vi "Read Events.vi"(8 "error in (no error)":errorcluster, 11 "Engine in":refnum<class "Engine.lvclass">) -> (0 "error out":errorcluster, 2 "Events":T1, 3 "Engine out":refnum<class "Engine.lvclass">)   [LabVIEW 2023, in "Engine.lvlib" / "Engine.lvclass"]
uses:
  Library/Engine.lvclass
  Custom Controls/Events.ctl
  Custom Controls/SystemEvents.ctl
  Custom Controls/Faults.ctl
  Custom Controls/Status.ctl
  Custom Controls/OtherEvents.ctl
  Custom Controls/AbstractMessage.ctl
  Library/Engine.lvclass/Engine.ctl
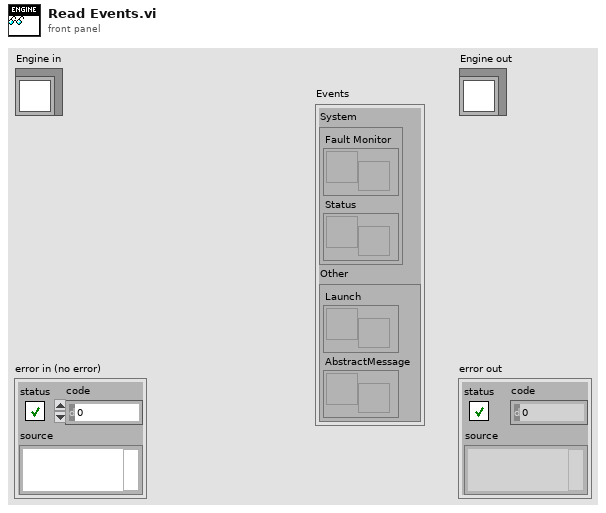
[diagram p1: front panel]
types:
  T1 = typedef "Engine.lvlib/Engine.lvclass/Events.ctl" = cluster{"System":T2, "Other":T3}
  T2 = typedef "Engine.lvlib/Engine.lvclass/SystemEvents.ctl" = cluster{"Fault Monitor":refnum<user-event>, "Status":refnum<user-event>}
  T3 = typedef "Engine.lvlib/Engine.lvclass/OtherEvents.ctl" = cluster{"Launch":refnum<user-event>, "AbstractMessage":refnum<user-event>}
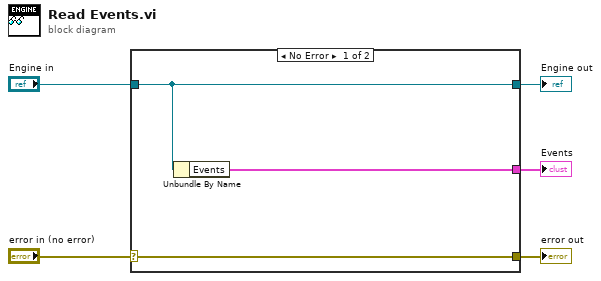
[diagram p0: block diagram]
diagram:
  n1 = case shown="No Error" "error in (no error)" {
    selector: "error in (no error)" -> [w8 w9]
    tunnel: [w8 w9] -> w4
    tunnel: [w7 w10] -> w2
    tunnel: "Engine in" -> [w7 w10]
    tunnel: [w6 _] -> w1
    frame No Error {
      n2 = Unbundle By Name(w7) -> ("Events"=w6:T1)
    }
    frame Error {
    }
  }
  "error out" <- w4
  "Engine out" <- w2
  "Events" <- w1
